vi "EditConnect.vi"(11 "ConnectConfig in":T1={"IP Address"="", "Port"=102, "Timeout"=5000}) -> (3 "ConnectConfig out":T1={"IP Address"="", "Port"=102, "Timeout"=5000})   [LabVIEW 2025, in "PLC_Module.lvlib" / "PLC_Module.lvclass"]
uses:
  PLC_Module.lvclass
  PLC_Connect_Config.ctl
panel:
  in  "Cancel":bool
  in  "OK":bool
  in  "ConnectConfig":T1={"IP Address"="", "Port"=102, "Timeout"=5000}
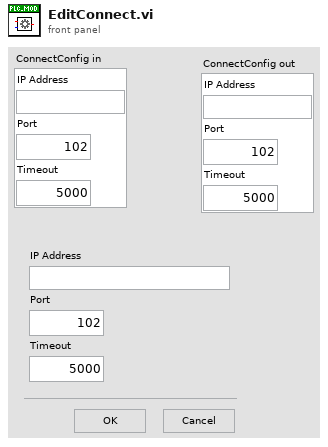
[diagram p1: front panel]
types:
  T1 = typedef "PLC_Module.lvlib/PLC_Module.lvclass/PLC_Connect_Config.ctl" = cluster{"IP Address":string, "Port":u16, "Timeout":i32}
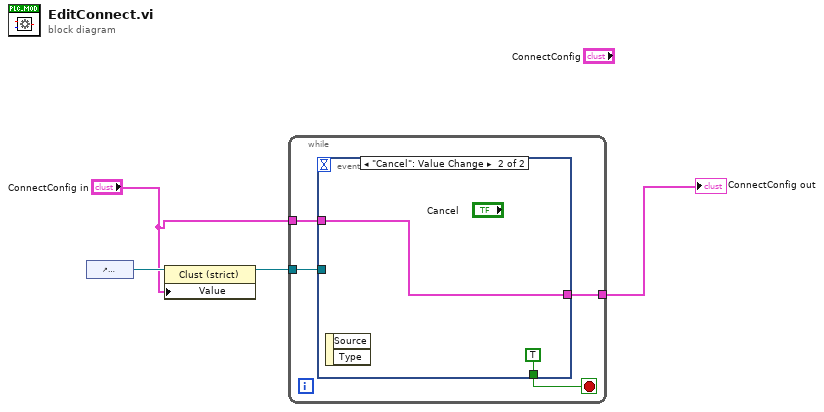
[diagram p0: block diagram]
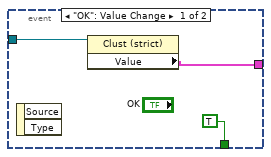
[diagram p2: hidden frame]
diagram:
  n1 = control-ref of="ConnectConfig"() -> (w4:refnum<vi>)
  n2 = property class="Clust (strict)"(reference=w4, "Value"="ConnectConfig in") -> (reference out=w3:refnum<vi>)  [unwired: 1 in, 1 out]
  n3 = while {
    tunnel: w3 -> [w8]
    tunnel: [w6] -> w2
    tunnel: "ConnectConfig in" -> [w5]
    stop <- w7 stop-if-true
    n4 = event shown="[1] \"Cancel\": Value Change" {
      selector: _ -> [_ _]
      dyn-events: _ -> [_ _]
      timeout: _ -> [_ _]
      tunnel: w8 -> [w11 _]
      tunnel: [TRUE TRUE] -> w7
      tunnel: [w9 w13] -> w6
      tunnel: w5 -> [_ w13]
      event "OK": Value Change {
        n5 = event-data() -> ()  [unwired: 1 in, 2 out]
        n6 = property class="Clust (strict)"(reference=w11) -> ("Value"=w9:T1)  [unwired: 1 in, 2 out]
      }
      event "Cancel": Value Change {
        n7 = event-data() -> ()  [unwired: 1 in, 2 out]
      }
    }
  }
  "ConnectConfig out" <- w2
